vi "CreateReferences.vi"(8 "error in (no error)":errorcluster, 11 "Connection in":refnum<class "Connection.lvclass">) -> (0 "error out":errorcluster, 3 "Connection out":refnum<class "Connection.lvclass">)   [LabVIEW 2013, in "MQTT_Connection.lvlib" / "Connection.lvclass"]
uses:
  Connection.lvclass
  Connection.lvclass/Connection.ctl
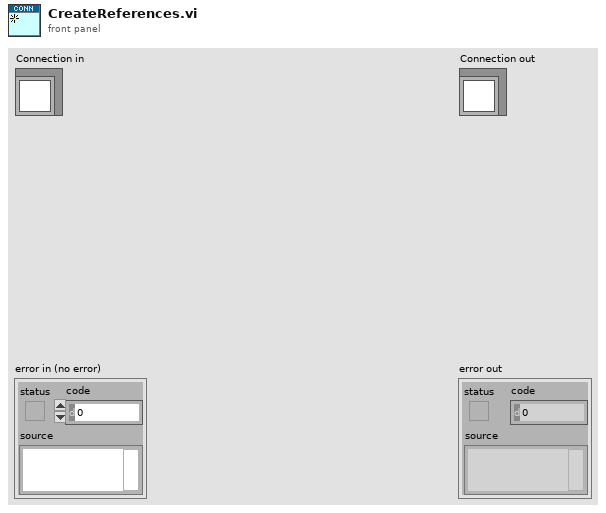
[diagram p1: front panel]
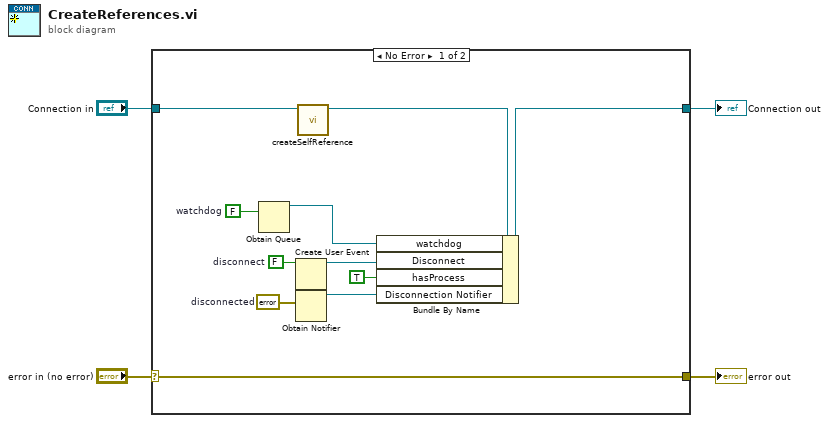
[diagram p0: block diagram]
diagram:
  n1 = case shown="No Error" "error in (no error)" {
    selector: "error in (no error)" -> [w15 w17]
    tunnel: [w15 w17] -> w3
    tunnel: [w8 w16] -> w1
    tunnel: "Connection in" -> [w6 w16]
    frame No Error {
      w9 = errorcluster {"status"=FALSE, "code"=0, "source"=""}  # disconnected
      w13 = FALSE  # disconnect
      w14 = FALSE  # watchdog
      n2 = Obtain Queue(element data type=w14) -> (queue out=w7:refnum<queue>)  [unwired: 4 in, 2 out]
      n3 = Create User Event(user event datatype=w13) -> (user event=w12:refnum<user-event>)  [unwired: 1 in, 1 out]
      n4 = Obtain Notifier(notification data type=w9) -> (notifier out=w10:refnum<notifier>)  [unwired: 3 in, 2 out]
      n5 = call "createSelfReference.vi"("Connection in"=w6) -> ("Connection out"=w5:refnum<class "Connection.lvclass">)  [unwired: 9 in, 1 out]
      n6 = Bundle By Name(cluster=w5, "watchdog"=w7, "Disconnect"=w12, "hasProcess"=TRUE, "Disconnection Notifier"=w10) -> (w8:refnum<class "Connection.lvclass">)
    }
    frame Error {
    }
  }
  "error out" <- w3
  "Connection out" <- w1
